vi "Stop Acquisition and Logging.vi"(8 "error in (no error)":errorcluster caption="错误输入（无错误）", 11 "FPGA VI Reference":T1 caption="FPGA VI引用") -> (0 "error out":errorcluster caption="错误输出", 3 "Stop FPGA Timeout?":bool caption="停止FPGA超时？")   [LabVIEW 2013]
doc: "本VI发送停止命令至FPGA采集循环，并等待循环已停止的确认信息。本VI也清空UI数据缓冲区，因此后续采集将不会读取旧数据。"
uses:
  controls/FPGA VI Reference.ctl
  <vilib>/rvi/interface/common/niFpgaWaitOnOcc.vi
  <vilib>/Utility/error.llb/Error Cluster From Error Code.vi
  <vilib>/rvi/errors/niLvFpgaAdjustHostInterfaceError.vi
  <vilib>/FPGAPlugInAG/cRIO-9074/niLvFpga_Close_cRIO-9074.vi
  <vilib>/rvi/interface/nirviReadWriteControl/nirviReadWriteControl.xnode
  FPGA Bitfiles/LabVIEWFPGAWavef_FPGA_FPGAMain_vTbN89OLNVY.lvbitx
  FPGA Main.vi
  <vilib>/rvi/interface/nirviMethod/nirviMethod.xnode
  <vilib>/rvi/interface/nirviCloseFPGA/nirviCloseFPGA.xnode
  NiFpgaLv.dll
  <vilib>/FPGAPlugInAG/cRIO-9074/niLvFpga_ReadFifo_cRIO-9074.vi
  <vilib>/rvi/errors/niLvFpgaMergeErrorWithErrorCode.vi
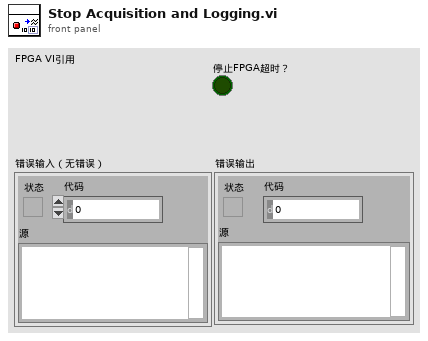
[diagram p1: front panel]
types:
  T1 = typedef "FPGA VI Reference.ctl" = refnum<k20>
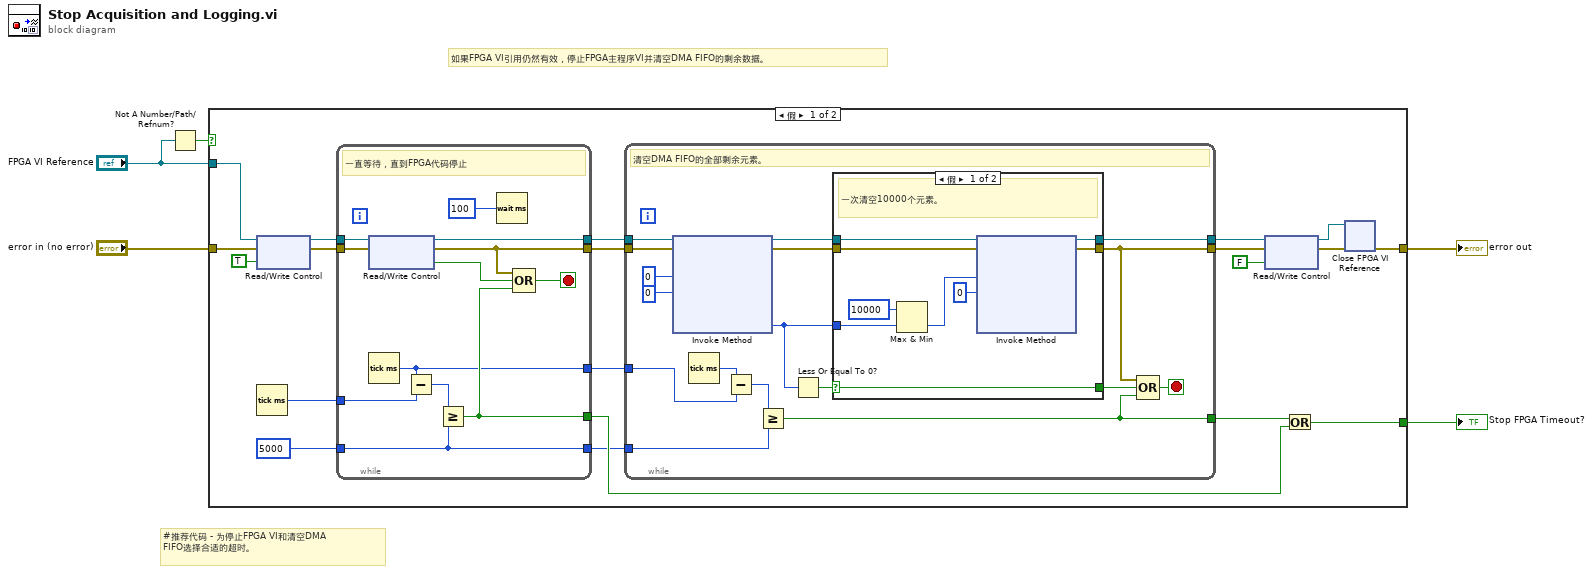
[diagram p0: block diagram]
diagram:
  # "#推荐代码 - 为停止FPGA VI和清空DMA FIFO选择合适的超时。"
  # "如果FPGA VI引用仍然有效，停止FPGA主程序VI并清空DMA FIFO的剩余数据。"
  n1 = Not A Number/Path/Refnum?(number/path/refnum="FPGA VI Reference") -> (NaN/Path/Refnum?=w2:bool)
  n2 = case shown="假" w2 {
    tunnel: [w11 w67] -> w5
    tunnel: "FPGA VI Reference" -> [w10 _]
    tunnel: "error in (no error)" -> [w9 w67]
    tunnel: [w7 _] -> w1
    frame False {
      n3 = xnode "Read/Write Control"("FPGA VI引用输入"=w10, "错误输入"=w9, "Stop"=TRUE) -> ("FPGA VI引用输出"=w23:T1, "错误输出"=w22:errorcluster)
      n4 = Tick Count (ms)() -> (millisecond timer value=w17:u32)
      n5 = while {
        tunnel: w23 -> [w66]
        tunnel: w22 -> [w65]
        tunnel: [w63] -> w21
        tunnel: [w56] -> w20
        tunnel: w17 -> [w62]
        tunnel: [w58] -> w15
        tunnel: [w57] -> w14
        tunnel: u32 5000 ("y") -> [w55]
        tunnel: [w55] -> w6
        stop <- w60 stop-if-true
        # "一直等待，直到FPGA代码停止"
        n6 = xnode "Read/Write Control"("FPGA VI引用输入"=w66, "错误输入"=w65) -> ("FPGA VI引用输出"=w63:T1, "错误输出"=w56:errorcluster, "Finished"=w59:bool)
        n7 = Tick Count (ms)() -> (millisecond timer value=w57:u32)
        n8 = Subtract(x=w57, y=w62) -> (x-y=w61:u32)
        n9 = Greater Or Equal?(x=w61, y=w55) -> (x >= y?=w58:bool)
        n10 = Wait (ms)(milliseconds to wait=u32 100) -> ()  [unwired: 1 out]
        n11 = Compound Arithmetic op=OR(w56, w59, w58) -> (w60:bool)
      }
      n12 = while {
        tunnel: [w39] -> w19
        tunnel: [w27] -> w18
        tunnel: w21 -> [w37]
        tunnel: w20 -> [w36]
        tunnel: w14 -> [w30]
        tunnel: [w29] -> w16
        tunnel: w6 -> [w28]
        stop <- w34 stop-if-true
        # "清空DMA FIFO的全部剩余元素。"
        n13 = xnode "Invoke Method"("FPGA VI引用输入"=w37, "错误输入"=w36, "元素数量"=u32 0 ("Number of Elements"), "超时(ms)"=0 ("Timeout (ms)")) -> ("FPGA VI引用输出"=w42:T1, "错误输出"=w41:errorcluster, "剩余元素"=w35:u32)  [unwired: 1 out]
        n14 = Tick Count (ms)() -> (millisecond timer value=w31:u32)
        n15 = Subtract(x=w31, y=w30) -> (x-y=w32:u32)
        n16 = Greater Or Equal?(x=w32, y=w28) -> (x >= y?=w29:bool)
        n17 = Less Or Equal To 0?(x=w35) -> (x <= 0?=w33:bool)
        n18 = case shown="假" w33 {
          selector: w33 -> [w46 w52]
          tunnel: w42 -> [w51 w54]
          tunnel: w41 -> [w50 w53]
          tunnel: [w48 w54] -> w39
          tunnel: [w47 w53] -> w27
          tunnel: w35 -> [w44 _]
          tunnel: [w46 w52] -> w26
          frame False {
            # "一次清空10000个元素。"
            n19 = Max & Min(x=u32 10000, y=w44) -> (min(x,y)=w43:u32)  [unwired: 1 out]
            n20 = xnode "Invoke Method"("FPGA VI引用输入"=w51, "错误输入"=w50, "元素数量"=w43, "超时(ms)"=0 ("Timeout (ms)")) -> ("FPGA VI引用输出"=w48:T1, "错误输出"=w47:errorcluster)  [unwired: 2 out]
          }
          frame True {
            # "缓冲区为空"
          }
        }
        n21 = Compound Arithmetic op=OR(w27, w26, w29) -> (w34:bool)
      }
      n22 = xnode "Read/Write Control"("FPGA VI引用输入"=w19, "错误输入"=w18, "Stop"=FALSE) -> ("FPGA VI引用输出"=w13:T1, "错误输出"=w12:errorcluster)
      n23 = Or(x=w16, y=w15) -> (x .or. y?=w7:bool)
      n24 = xnode "Close FPGA VI Reference"("FPGA VI引用输入"=w13, "错误输入"=w12) -> ("错误输出"=w11:errorcluster)
    }
    frame True {
    }
  }
  "error out" <- w5
  "Stop FPGA Timeout?" <- w1
